vi "e.gate HighSpeedPort Decode Interface Diagnostic.vi"(8 "error in":errorcluster, 10 "IsBigEndian":i32, 11 "Binary Data in":u8[](array[numeric])) -> (0 "error out":errorcluster, 1 "Error Count":i32[](array[numeric]), 2 "Cycles Count":i32[](array[numeric]), 3 "Remaining Binary Data":u8[](array[numeric]), 4 "DeltaTimeS":dbl[](array[numeric]), 5 "Interface Index":i16[](array[numeric]), 7 "Interface Kind":string[](array[string]))   [LabVIEW 2016]
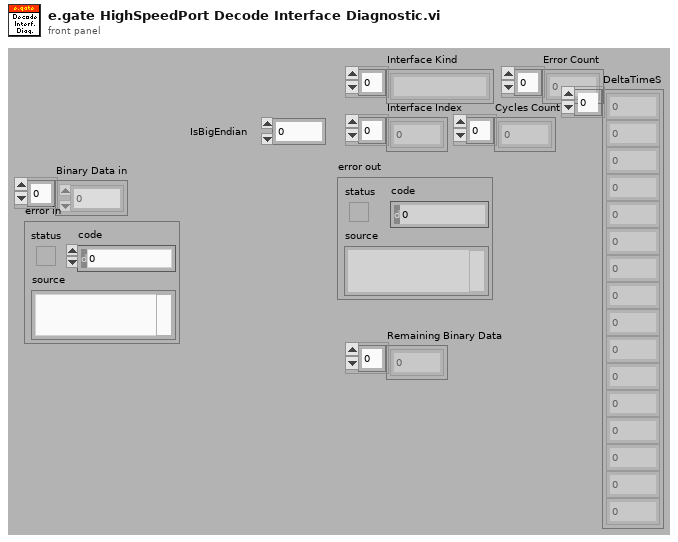
[diagram p1: front panel]
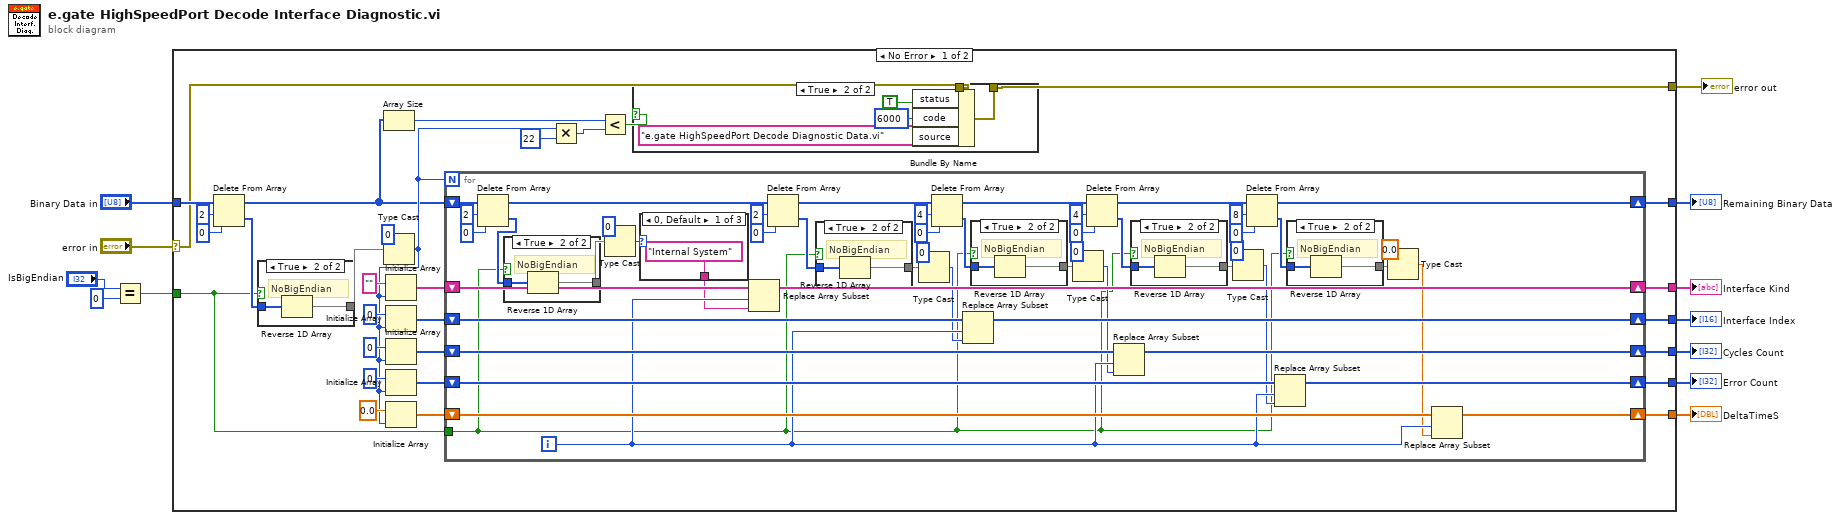
[diagram p0: block diagram]
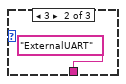
[diagram p9: hidden frame]
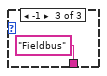
[diagram p10: hidden frame]
diagram:
  n1 = Equal?(x="IsBigEndian", y=0) -> (x = y?=w1:bool)
  n2 = case shown="No Error" "error in" {
    selector: "error in" -> [w21 w120]
    tunnel: "Binary Data in" -> [w40 _]
    tunnel: [w29 _] -> w9
    tunnel: [w28 _] -> w8
    tunnel: [w27 _] -> w7
    tunnel: [w26 _] -> w6
    tunnel: [w25 _] -> w5
    tunnel: [w24 _] -> w4
    tunnel: [w20 w120] -> w10
    tunnel: w1 -> [w13 _]
    frame No Error {
      n3 = Delete From Array(array=w40, length=2 ("Länge"), index=0 ("Index")) -> (deleted portion=w15:u8[], array with subset deleted=w16:u8[])
      n4 = case shown="True" w13 {
        tunnel: w15 -> [w44 w46]
        tunnel: [w44 w45] -> w14
        frame False {
        }
        frame True {
          # "NoBigEndian"
          n5 = Reverse 1D Array(array=w46) -> (reversed array=w45:u8[])
        }
      }
      n6 = Array Size(array=w16) -> (size(s)=w22:i32)
      n7 = Type Cast(type=i16 0, x=w14) -> (*(type *) &x=w19:i16)
      n8 = Initialize Array("", w19) -> (w39:string[])
      n9 = Initialize Array(i16 0, w19) -> (w35:i16[])
      n10 = Initialize Array(0 ("Element"), w19) -> (w34:i32[])
      n11 = Initialize Array(0 ("Element"), w19) -> (w31:i32[])
      n12 = Initialize Array(0.0 ("Element"), w19) -> (w30:dbl[])
      n13 = for {
        N: w19 -> [_]
        shift-right: [w87] -> w24
        shift-left: w16 -> [w86]
        shift-right: [w84] -> w29
        shift-left: w39 -> [w85]
        shift-right: [w82] -> w28
        shift-left: w35 -> [w83]
        shift-right: [w80] -> w27
        shift-left: w34 -> [w81]
        shift-right: [w78] -> w26
        shift-left: w31 -> [w79]
        shift-right: [w76] -> w25
        shift-left: w30 -> [w77]
        tunnel: w13 -> [w54]
        i -> [w75]
        n14 = Delete From Array(array=w86, length=2 ("Länge"), index=0 ("Index")) -> (deleted portion=w63:u8[], array with subset deleted=w97:u8[])
        n15 = case shown="True" w54 {
          tunnel: w63 -> [w114 w116]
          tunnel: [w114 w115] -> w62
          frame False {
          }
          frame True {
            # "NoBigEndian"
            n16 = Reverse 1D Array(array=w116) -> (reversed array=w115:u8[])
          }
        }
        n17 = Type Cast(type=i16 0, x=w62) -> (*(type *) &x=w65:i16)
        n18 = case shown="0, Default" w65 {
          tunnel: ["Internal System" ("Neues Element/Teilarray") "ExternalUART" ("Neues Element/Teilarray") "Fieldbus" ("Neues Element/Teilarray")] -> w64
          frame 0, Default {
          }
          frame 3 {
          }
          frame -1 {
          }
        }
        n19 = Replace Array Subset(array=w85, new element=w64, index=w75) -> (w84:string[])
        n20 = Delete From Array(array=w97, length=2 ("Länge"), index=0 ("Index")) -> (deleted portion=w61:u8[], array with subset deleted=w90:u8[])
        n21 = case shown="True" w54 {
          tunnel: w61 -> [w111 w113]
          tunnel: [w111 w112] -> w60
          frame False {
          }
          frame True {
            # "NoBigEndian"
            n22 = Reverse 1D Array(array=w113) -> (reversed array=w112:u8[])
          }
        }
        n23 = Type Cast(type=i16 0, x=w60) -> (*(type *) &x=w70:i16)
        n24 = Delete From Array(array=w90, length=4 ("Länge"), index=0 ("Index")) -> (deleted portion=w59:u8[], array with subset deleted=w89:u8[])
        n25 = Replace Array Subset(array=w83, new element=w70, index=w75) -> (w82:i16[])
        n26 = case shown="True" w54 {
          tunnel: w59 -> [w108 w110]
          tunnel: [w108 w109] -> w58
          frame False {
          }
          frame True {
            # "NoBigEndian"
            n27 = Reverse 1D Array(array=w110) -> (reversed array=w109:u8[])
          }
        }
        n28 = Type Cast(type=0, x=w58) -> (*(type *) &x=w69:i32)
        n29 = Delete From Array(array=w89, length=4 ("Länge"), index=0 ("Index")) -> (deleted portion=w57:u8[], array with subset deleted=w88:u8[])
        n30 = Replace Array Subset(array=w81, new element=w69, index=w75) -> (w80:i32[])
        n31 = case shown="True" w54 {
          tunnel: w57 -> [w105 w107]
          tunnel: [w105 w106] -> w56
          frame False {
          }
          frame True {
            # "NoBigEndian"
            n32 = Reverse 1D Array(array=w107) -> (reversed array=w106:u8[])
          }
        }
        n33 = Type Cast(type=0, x=w56) -> (*(type *) &x=w68:i32)
        n34 = Delete From Array(array=w88, length=8 ("Länge"), index=0 ("Index")) -> (deleted portion=w55:u8[], array with subset deleted=w87:u8[])
        n35 = Replace Array Subset(array=w79, new element=w68, index=w75) -> (w78:i32[])
        n36 = case shown="True" w54 {
          tunnel: w55 -> [w102 w104]
          tunnel: [w102 w103] -> w53
          frame False {
          }
          frame True {
            # "NoBigEndian"
            n37 = Reverse 1D Array(array=w104) -> (reversed array=w103:u8[])
          }
        }
        n38 = Type Cast(type=0.0, x=w53) -> (*(type *) &x=w67:dbl)
        n39 = Replace Array Subset(array=w77, new element=w67, index=w75) -> (w76:dbl[])
      }
      n40 = Multiply(x=w19, y=i16 22) -> (x*y=w17:i16)
      n41 = Less?(x=w22, y=w17) -> (x < y?=w23:bool)
      n42 = case shown="True" w23 {
        tunnel: w21 -> [w47 w52]
        tunnel: [w47 w51] -> w20
        frame False {
        }
        frame True {
          n43 = Bundle By Name(cluster=w52, "status"=TRUE, "code"=6000, "source"="e.gate HighSpeedPort Decode Diagnostic Data.vi") -> (w51:errorcluster)
        }
      }
    }
    frame Error {
    }
  }
  "error out" <- w10
  "Interface Kind" <- w9
  "Interface Index" <- w8
  "Cycles Count" <- w7
  "Error Count" <- w6
  "DeltaTimeS" <- w5
  "Remaining Binary Data" <- w4
